vi "DCPower_CurrentLimit&MeasureRecordReadout.vi"(8 "error in (no error)":errorcluster, 10 "Active Channel Numbers Array":string[](array[string]), 11 "IVI Refnum in":refnum<k15>) -> (0 "error out":errorcluster, 1 "Active Channel Measure Record Delta Time Array":dbl[](array[numeric]), 2 "Active Channel Current Limit Array":dbl[](array[numeric]), 3 "IVI Refnum out":refnum<k15>)   [LabVIEW 2019]
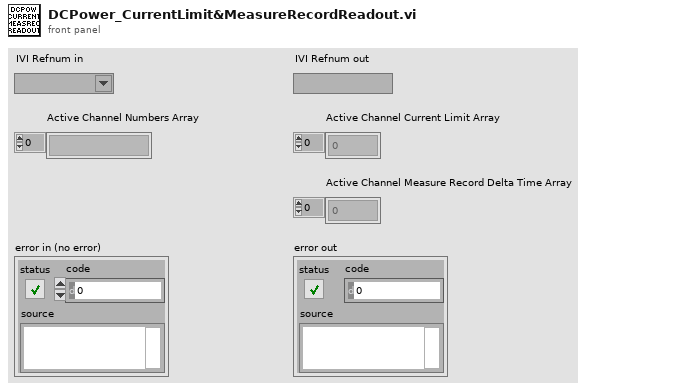
[diagram p1: front panel]
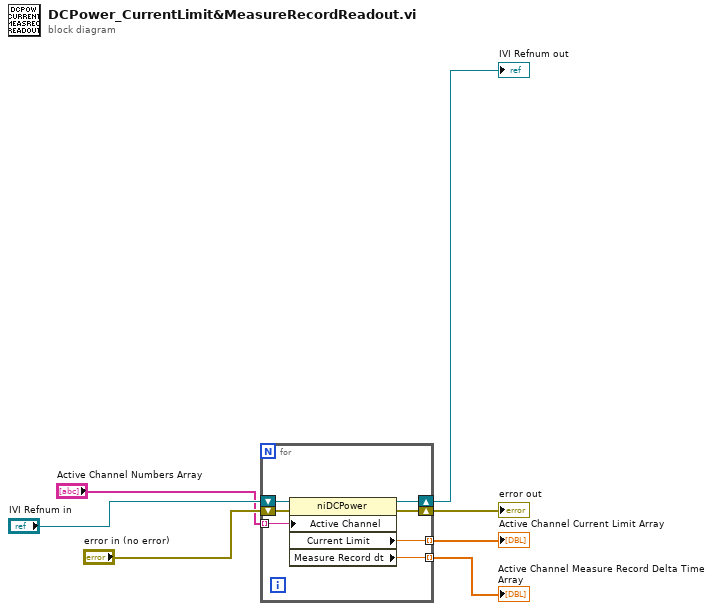
[diagram p0: block diagram]
diagram:
  n1 = for {
    tunnel: "Active Channel Numbers Array" -> [w14] mode=indexing
    shift-right: [w11] -> w4
    shift-left: "error in (no error)" -> [w12]
    shift-right: [w10] -> w5
    shift-left: "IVI Refnum in" -> [w13]
    tunnel: [w9] -> w7 mode=indexing
    tunnel: [w8] -> w6 mode=indexing
    n2 = property class="niDCPower"(reference=w13, error in=w12, "Active Channel"=w14) -> (reference out=w10:refnum<k15>, error out=w11:errorcluster, "Current Limit"=w9:dbl, "Measure Record dt"=w8:dbl)
  }
  "Active Channel Current Limit Array" <- w7
  "Active Channel Measure Record Delta Time Array" <- w6
  "IVI Refnum out" <- w5
  "error out" <- w4
